vi "MathCad_Easy_Numeric_Set_Var.vi"(8 "error in (no error)":errorcluster, 9 "Data In":cluster{"value":dbl, "New Variable Name":string} {"value" format="%.2f"}, 11 "Mathcad Reference":T1) -> (0 "error out":errorcluster, 3 "Mathcad Reference":T1)   [LabVIEW 2015]
doc: "Sets a Numeric value in Mathcad. You can also use this VI to reset a variable that has already been set once. It is only dependent upon the variable name. The variable won't appear in the Mathcad worksheet, but is defined at the very beginning of the worksheet.\nInputs \n Wrksht Ref--ActiveX Reference to Mathcad Worksheet Class\n Data In--Name and Value of Variable to Set\n Cluster (2 elements)\n Value (Double)\n New Variable Name(String)\nOutputs \n Wrksht Ref--ActiveX Reference to Mathcad Worksheet Class"
uses:
  Mathcad Reference.ctl
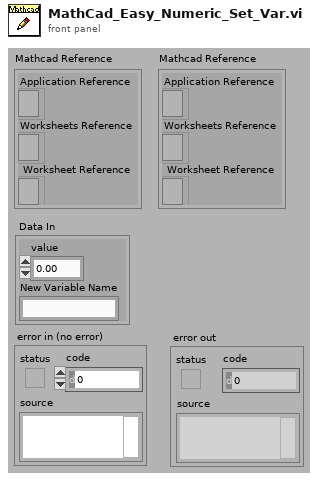
[diagram p1: front panel]
types:
  T1 = typedef "Mathcad Reference.ctl" = cluster{"Application Reference":refnum<k7>, "Worksheets Reference":refnum<k7>, " Worksheet Reference":refnum<k7>}
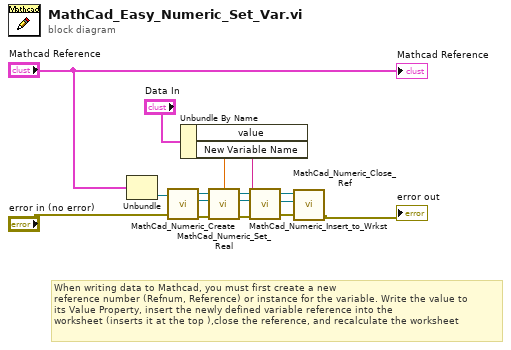
[diagram p0: block diagram]
diagram:
  # "When writing data to Mathcad, you must first create a new \nreference number (Refnum, Reference) or instance for the variable. Write the value to\nits Value Property, insert the newly defined variable reference into the\nworksheet (inserts it at the top ),close the reference, and recalculate the worksheet"
  n1 = Unbundle("Mathcad Reference") -> ("Worksheet Reference"=w2:refnum<k7>)  [unwired: 2 out]
  n2 = call "MathCad_Numeric_Create.vi"("error in (no error)"="error in (no error)", "Worksheet Reference In"=w2) -> ("error out"=w13:errorcluster, "Mathcad.INumericValue Reference Out"=w14:refnum<k7>, "Worksheet Reference Out"=w15:refnum<k7>)  [unwired: 1 in]
  n3 = Unbundle By Name("Data In") -> ("value"=w7:dbl, "New Variable Name"=w8:string)
  n4 = call "MathCad_Numeric_Set_Real.vi"("Worksheet Reference In"=w15, "Real"=w7, "Mathcad.INumericValue Refnum In"=w14, "error in"=w13) -> ("Worksheet Reference Out"=w11:refnum<k7>, "Mathcad.INumericValue Refnum Out"=w10:refnum<k7>, "error out"=w9:errorcluster)  [unwired: 9 in]
  n5 = call "MathCad_Numeric_Insert_to_Wrkst.vi"("error out 2"=w9, "New Variable Name"=w8, "Mathcad.INumericValue Ref In"=w10, "Wrksht Ref In"=w11) -> ("error out"=w4:errorcluster, "Mathcad.INumericValue Ref Out"=w6:refnum<k7>, "Wrksht Ref Out"=w5:refnum<k7>)
  n6 = call "MathCad_Numeric_Close_Ref.vi"("error in"=w4, "Mathcad.INumericValue Reference"=w6, "IMathcadWorksheet Reference"=w5) -> ("error out"=→"error out":errorcluster)  [unwired: 2 in, 1 out]
  "Mathcad Reference" <- "Mathcad Reference"
